vi "Pagina parametri.vi"() -> (6 "pagina out":i16)   [LabVIEW 2022 SP3]
uses:
  Labview/Globali.vi
panel:
  in  "230. 0":sgl min=0 format="%.2f"
  in  "226. 0":sgl min=0 format="%.2f"
  in  "Azzeramento \ntorsiometro (V)":sgl min=0 format="%.2f"
  in  "Carica da file":bool
  in  "Salva":bool
  in  "stop":bool
  out "Indicazioni":string
  out "Prodotto":string
  out "Testo allarmi":string caption="ALLARMI"
  out "Testo fase collaudo":string caption="FASE COLLAUDO"
  out "Testo segnalazioni":string caption="SEGNALAZIONI"
  out "Testo messaggi":string caption="MESSAGGI"
  out "Tipo pagina":string
  out "Picture":picture
  out "Versione SW":dbl=1.0 format="%.2f"
  out "Linea":string="CENTAURO"
  in  "8. 0":i16 min=0
  in  "12. 0":sgl min=0 format="%.2f"
  in  "16. 0":i16 min=0
  in  "22. 0":sgl min=0 format="%.2f"
  in  "26. 0":sgl min=0 format="%.2f"
  in  "32. 0":sgl min=0 format="%.2f"
  in  "36. 0":sgl min=0 format="%.2f"
  in  "44. 0":i16 min=0
  in  "50. 0":i16 min=0
  in  "56. 0":i16 min=0
  in  "62. 0":i16 min=0
  in  "68. 0":i16 min=0
  in  "72. 0":sgl min=0 format="%.2f"
  in  "76. 0":sgl min=0 format="%.2f"
  in  "80. 0":sgl min=0 format="%.2f"
  in  "84. 0":i16 min=0
  in  "88. 0":sgl min=0 format="%.2f"
  in  "92. 0":sgl min=0 format="%.2f"
  in  "96. 0":sgl min=0 format="%.2f"
  in  "100. 0":i16 min=0
  in  "104. 0":sgl min=0 format="%.2f"
  in  "108. 0":sgl min=0 format="%.2f"
  in  "112. 0":sgl min=0 format="%.2f"
  in  "116. 0":i16 min=0
  in  "120. 0":sgl min=0 format="%.2f"
  in  "124. 0":sgl min=0 format="%.2f"
  in  "128. 0":sgl min=0 format="%.2f"
  in  "134. 0":sgl min=0 format="%.2f"
  in  "138. 0":sgl min=0 format="%.2f"
  in  "144. 0":i16 min=0
  in  "148. 0":i16 min=0
  in  "154. 0":i16 min=0
  in  "160. 0":sgl min=0 format="%.2f"
  in  "164. 0":sgl min=0 format="%.2f"
  in  "168. 0":sgl min=0 format="%.2f"
  in  "172. 0":i16 min=0
  in  "176. 0":sgl min=0 format="%.2f"
  in  "180. 0":sgl min=0 format="%.2f"
  in  "184. 0":sgl min=0 format="%.2f"
  in  "190. 0":sgl min=0 format="%.2f"
  in  "194. 0":sgl min=0 format="%.2f"
  in  "200. 0":i16 min=0
  in  "206. 0":i16 min=0
  in  "212. 0":i16 min=0
  in  "20. 0":u16
  in  "30. 0":u16
  in  "40. 0":u16
  in  "42. 0":u16
  in  "48. 0":u16
  in  "54. 0":u16
  in  "60. 0":u16
  in  "66. 0":u16
  in  "132. 0":u16
  in  "142. 0":u16
  in  "152. 0":u16
  in  "158. 0":u16
  in  "188. 0":u16
  in  "198. 0":u16
  in  "204. 0":u16
  in  "210. 0":u16
  in  "216. 0":u16
  in  "218. 0":u16
  in  "NOME PRODOTTO":string
  out "error out":errorcluster
  in  "error in":errorcluster
  # "RISCALDAMENTO"
  # "FUNZIONAMENTO"
  # "Temperatura olio RP riscaldamento"
  # "Pressione ricircolo minima"
  # "Pressione gonfiaggio minima"
  # "Velocità motore riscaldamento"
  # "Pressione ricircolo massima"
  # "Pressione gonfiaggio massima"
  # "Tempo AAT riscaldamento"
  # "Velocità motore 1 funzionamento"
  # "Tempo stabilizzazione gonfiaggio"
  # "Pressione olio ricircolo minima"
  # "Temperatura olio 1 funzionamento"
  # "Vel. motore 4 funzionamento RP dx"
  # "K_VEL_MOT_MAN"
  # "Pressione olio ricircolo massima"
  # "Coppia 1 funzionamento minima"
  # "Velocità motore 4 funzionamento"
  # "Coppia 1 funzionamento massima"
  # "Tempo 4 funzionamento RP dx"
  # "Velocità motore 2 funzionamento"
  # "Vel. motore 4 funzionamento RP sx"
  # "INSERZIONE 1° ASSE"
  # "Temperatura olio 2 funzionamento"
  # "Tempo 4 funzionamento RP sx"
  # "Tempo pressurizzazione inserzione"
  # "Coppia 2 funzionamento minima"
  # "Temperatura olio 4 funzionamento"
  # "Pressurizzaz. inserz. asse minima"
  # "Coppia 2 funzionamento massima"
  # "Coppia 4 funzionamento minima"
  # "Pressurizzaz. inserz. asse massima"
  # "Velocità motore 3 funzionamento"
  # "Coppia 4 funzionamento massima"
  # "Tempo inserzione 1° asse"
  # "Temperatura olio 3 funzionamento"
  # "Velocità motore 5 funzionamento"
  # "Tempo disinserzione 1° asse"
  # "Coppia 3 funzionamento minima"
  # "Temperatura olio 5 funzionamento"
  # "Coppia 3 funzionamento massima"
  # "Coppia 5 funzionamento minima"
  # "Tempo gonfiaggio"
  # "Coppia 5 funzionamento massima"
  # "RODAGGIO"
  # "Perdita gonfiaggio"
  # "Velocità 1 motore rodaggio"
  # "PRESSURIZZAZIONE"
  # "PROT35"
  # "Tempo 1 rodaggio"
  # "Tempo pressurizzazione"
  # "Velocità motore PROT35"
  # "Velocità 2 motore rodaggio"
  # "Pressurizzazione minima"
  # "Tempo PROT35 sx"
  # "Tempo 2 rodaggio"
  # "Pressurizzazione massima"
  # "Tempo PROT35 dx"
  # "Velocità 3 motore rodaggio"
  # "Tempo stabilizzazione pressurizzaz."
  # "Tempo 3 rodaggio"
  # "Velocità pressurizzazione dx"
  # "Velocità 4 motore rodaggio"
  # "Tempo pressurizzazione dx"
  # "Tempo 4 rodaggio"
  # "Velocità pressurizzazione sx"
  # "Velocità 5 motore rodaggio"
  # "Tempo pressurizzazione sx"
  # "Temperatura olio rodaggio"
  # "Perdita pressurizzazione"
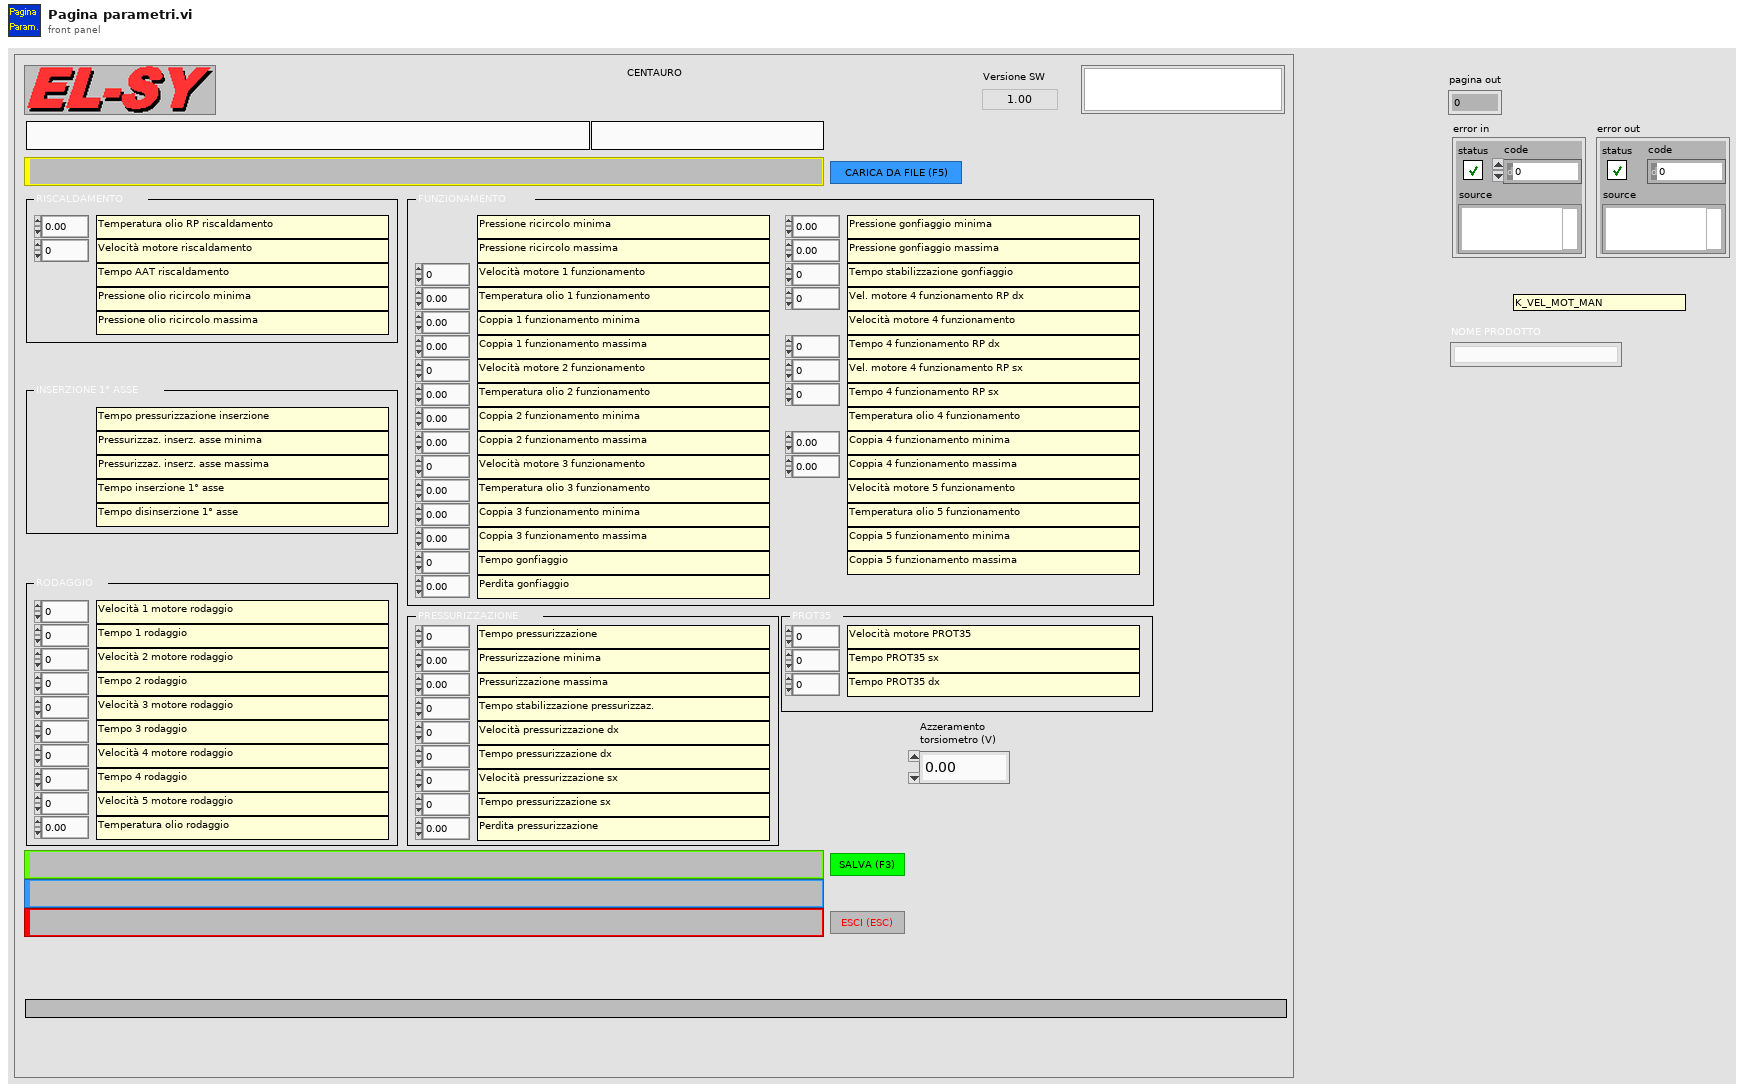
[diagram p1: front panel]
types:
  T1 = enum16{"open", "open or create", "create or replace", "create", "open (read only)"}
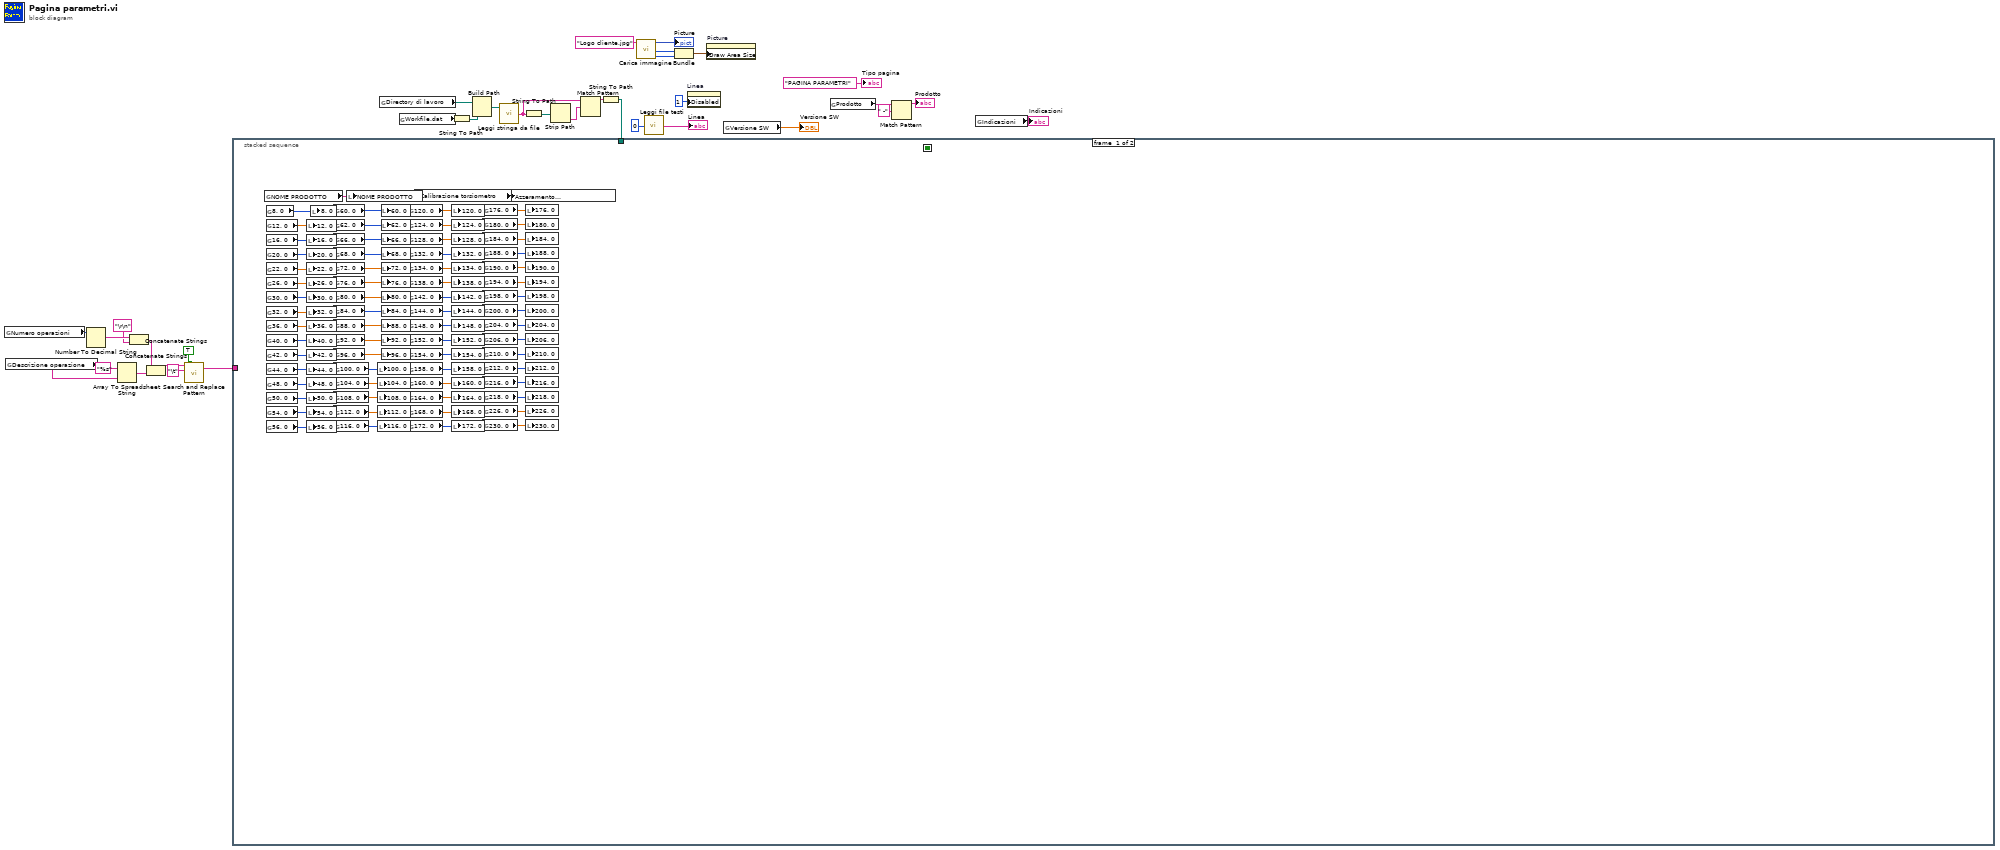
[diagram p0: block diagram]
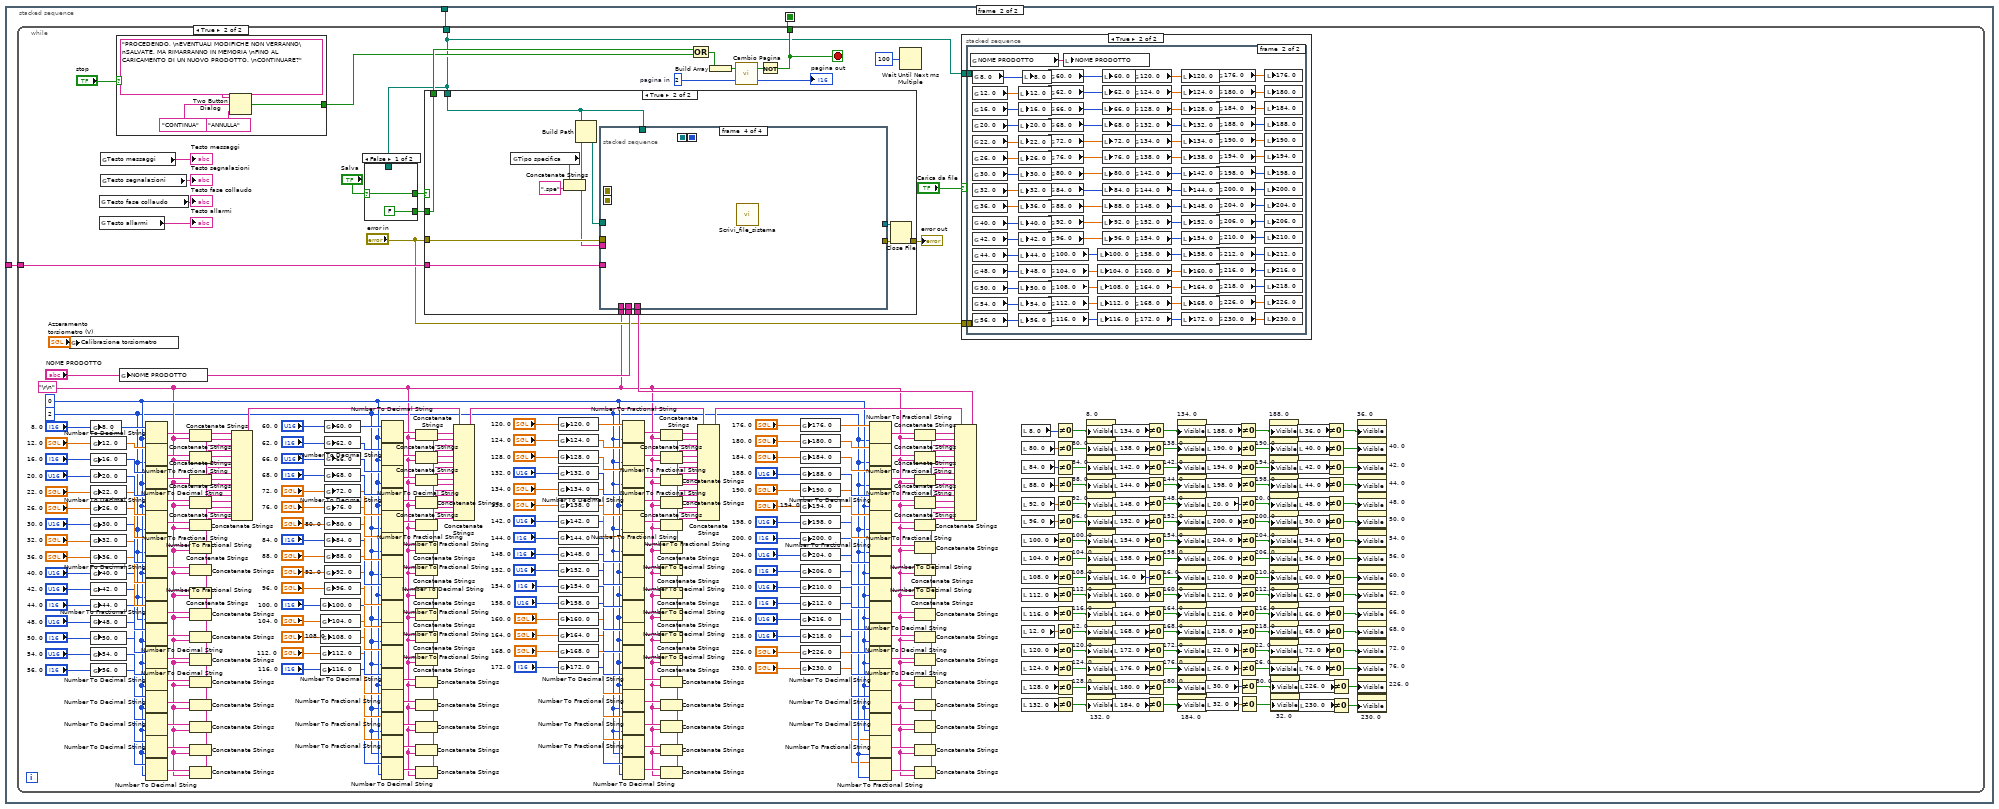
[diagram p2: hidden frame]
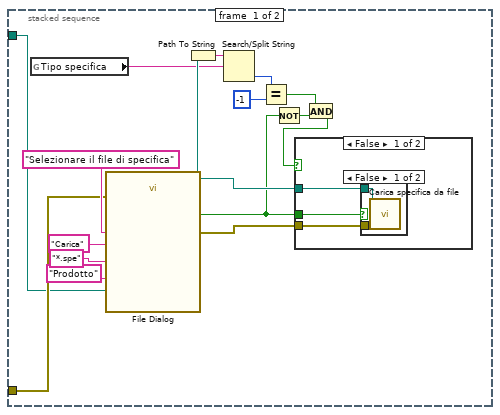
[diagram p4: hidden frame]
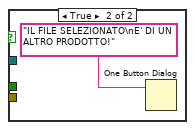
[diagram p6: hidden frame]
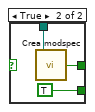
[diagram p8: hidden frame]
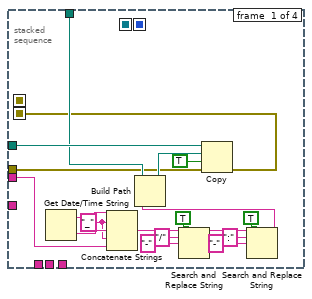
[diagram p10: hidden frame]
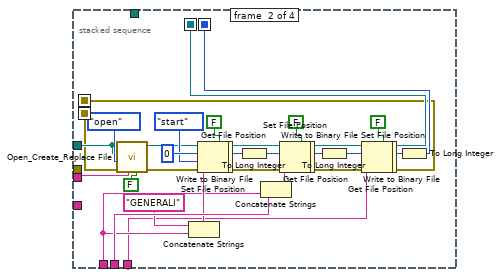
[diagram p11: hidden frame]
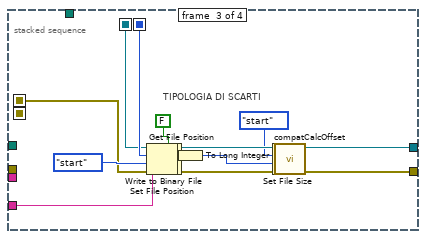
[diagram p12: hidden frame]
diagram:
  n1 = global read "Globali.vi" "Numero operazioni"() -> (w13:u16)
  n2 = global read "Globali.vi" "Descrizione operazione"() -> (w16:string[])
  n3 = Number To Decimal String(number=w13) -> (decimal integer string=w12:string)  [unwired: 1 in]
  n4 = Array To Spreadsheet String(array=w16, 3:"%s" ("format string")) -> (spreadsheet string=w15:string)  [unwired: 1 in]
  n5 = Concatenate Strings(w12, "\r\n" ("delimiter (Tab)")) -> (w11:string)
  n6 = Concatenate Strings(w11, w15) -> (w8:string)
  n7 = call <vilib>:"Search and Replace Pattern.vi"("string"=w8, "regular expression (\"\")"="\t" ("regular expression (\"\")"), "replace all? (F)"=TRUE) -> ("result string"=w9:string)  [unwired: 2 in, 1 out]
  n8 = global read "Globali.vi" "Directory di lavoro"() -> (w32:path)
  n9 = global read "Globali.vi" "Workfile.dat"() -> (w31:string)
  n10 = String To Path(string=w31) -> (path=w34:path)
  n11 = Build Path(base path=w32, name or relative path=w34) -> (appended path=w33:path)
  n12 = call "Leggi stringa da file.vi"("file path (dialog if empty)"=w33) -> ("character string"=w27:string)  [unwired: 5 in, 3 out]
  n13 = String To Path(string=w27) -> (path=w30:path)
  n14 = Strip Path(path=w30) -> (name=w29:string)  [unwired: 1 out]
  n15 = Match Pattern(string=w27, regular expression=w29) -> (before substring=w28:string)  [unwired: 1 in, 3 out]
  n16 = String To Path(string=w28) -> (path=w26:path)
  n17 = stacked-sequence {
    seq-local: [_ w102] -> [_ _]
    tunnel: w26 -> [_ w103]
    tunnel: w9 -> [_ w101]
    frame #0 {
      n18 = global read "Globali.vi" "NOME PRODOTTO"() -> (w100:string)
      n19 = global read "Globali.vi" "8. 0"() -> (w99:i16)
      n20 = global read "Globali.vi" "12. 0"() -> (w98:sgl)
      n21 = global read "Globali.vi" "16. 0"() -> (w97:i16)
      n22 = global read "Globali.vi" "20. 0"() -> (w96:u16)
      n23 = global read "Globali.vi" "22. 0"() -> (w95:sgl)
      n24 = global read "Globali.vi" "26. 0"() -> (w94:sgl)
      n25 = global read "Globali.vi" "30. 0"() -> (w93:u16)
      n26 = global read "Globali.vi" "32. 0"() -> (w92:sgl)
      n27 = global read "Globali.vi" "36. 0"() -> (w91:sgl)
      n28 = global read "Globali.vi" "40. 0"() -> (w90:u16)
      n29 = global read "Globali.vi" "42. 0"() -> (w89:u16)
      n30 = global read "Globali.vi" "44. 0"() -> (w88:i16)
      n31 = global read "Globali.vi" "48. 0"() -> (w87:u16)
      n32 = global read "Globali.vi" "50. 0"() -> (w86:i16)
      n33 = global read "Globali.vi" "54. 0"() -> (w85:u16)
      n34 = global read "Globali.vi" "56. 0"() -> (w84:i16)
      n35 = local write "12. 0"(w98) -> ()
      n36 = local write "16. 0"(w97) -> ()
      n37 = local write "20. 0"(w96) -> ()
      n38 = local write "22. 0"(w95) -> ()
      n39 = local write "26. 0"(w94) -> ()
      n40 = local write "30. 0"(w93) -> ()
      n41 = local write "32. 0"(w92) -> ()
      n42 = local write "36. 0"(w91) -> ()
      n43 = local write "40. 0"(w90) -> ()
      n44 = local write "42. 0"(w89) -> ()
      n45 = local write "44. 0"(w88) -> ()
      n46 = local write "48. 0"(w87) -> ()
      n47 = local write "50. 0"(w86) -> ()
      n48 = local write "54. 0"(w85) -> ()
      n49 = local write "56. 0"(w84) -> ()
      n50 = local write "8. 0"(w99) -> ()
      n51 = global read "Globali.vi" "60. 0"() -> (w83:u16)
      n52 = global read "Globali.vi" "62. 0"() -> (w82:i16)
      n53 = global read "Globali.vi" "66. 0"() -> (w81:u16)
      n54 = global read "Globali.vi" "68. 0"() -> (w80:i16)
      n55 = global read "Globali.vi" "72. 0"() -> (w79:sgl)
      n56 = global read "Globali.vi" "76. 0"() -> (w78:sgl)
      n57 = global read "Globali.vi" "80. 0"() -> (w77:sgl)
      n58 = global read "Globali.vi" "84. 0"() -> (w76:i16)
      n59 = global read "Globali.vi" "88. 0"() -> (w75:sgl)
      n60 = global read "Globali.vi" "92. 0"() -> (w74:sgl)
      n61 = global read "Globali.vi" "96. 0"() -> (w73:sgl)
      n62 = global read "Globali.vi" "100. 0"() -> (w72:i16)
      n63 = global read "Globali.vi" "104. 0"() -> (w71:sgl)
      n64 = global read "Globali.vi" "108. 0"() -> (w70:sgl)
      n65 = global read "Globali.vi" "112. 0"() -> (w69:sgl)
      n66 = global read "Globali.vi" "116. 0"() -> (w68:i16)
      n67 = local write "NOME PRODOTTO"(w100) -> ()
      n68 = local write "100. 0"(w72) -> ()
      n69 = local write "104. 0"(w71) -> ()
      n70 = local write "108. 0"(w70) -> ()
      n71 = local write "112. 0"(w69) -> ()
      n72 = local write "116. 0"(w68) -> ()
      n73 = local write "60. 0"(w83) -> ()
      n74 = local write "62. 0"(w82) -> ()
      n75 = local write "66. 0"(w81) -> ()
      n76 = local write "68. 0"(w80) -> ()
      n77 = local write "72. 0"(w79) -> ()
      n78 = local write "76. 0"(w78) -> ()
      n79 = local write "80. 0"(w77) -> ()
      n80 = local write "84. 0"(w76) -> ()
      n81 = local write "88. 0"(w75) -> ()
      n82 = local write "92. 0"(w74) -> ()
      n83 = local write "96. 0"(w73) -> ()
      n84 = global read "Globali.vi" "120. 0"() -> (w67:sgl)
      n85 = global read "Globali.vi" "124. 0"() -> (w66:sgl)
      n86 = global read "Globali.vi" "128. 0"() -> (w65:sgl)
      n87 = global read "Globali.vi" "132. 0"() -> (w64:u16)
      n88 = global read "Globali.vi" "134. 0"() -> (w63:sgl)
      n89 = global read "Globali.vi" "138. 0"() -> (w62:sgl)
      n90 = global read "Globali.vi" "142. 0"() -> (w61:u16)
      n91 = global read "Globali.vi" "144. 0"() -> (w60:i16)
      n92 = global read "Globali.vi" "148. 0"() -> (w59:i16)
      n93 = global read "Globali.vi" "152. 0"() -> (w58:u16)
      n94 = global read "Globali.vi" "154. 0"() -> (w57:i16)
      n95 = global read "Globali.vi" "158. 0"() -> (w56:u16)
      n96 = global read "Globali.vi" "160. 0"() -> (w55:sgl)
      n97 = global read "Globali.vi" "164. 0"() -> (w54:sgl)
      n98 = global read "Globali.vi" "168. 0"() -> (w53:sgl)
      n99 = global read "Globali.vi" "172. 0"() -> (w52:i16)
      n100 = global read "Globali.vi" "Calibrazione torsiometro"() -> (w37:sgl)
      n101 = local write "120. 0"(w67) -> ()
      n102 = local write "124. 0"(w66) -> ()
      n103 = local write "128. 0"(w65) -> ()
      n104 = local write "132. 0"(w64) -> ()
      n105 = local write "134. 0"(w63) -> ()
      n106 = local write "138. 0"(w62) -> ()
      n107 = local write "142. 0"(w61) -> ()
      n108 = local write "144. 0"(w60) -> ()
      n109 = local write "148. 0"(w59) -> ()
      n110 = local write "152. 0"(w58) -> ()
      n111 = local write "154. 0"(w57) -> ()
      n112 = local write "158. 0"(w56) -> ()
      n113 = local write "160. 0"(w55) -> ()
      n114 = local write "164. 0"(w54) -> ()
      n115 = local write "168. 0"(w53) -> ()
      n116 = local write "172. 0"(w52) -> ()
      n117 = global read "Globali.vi" "176. 0"() -> (w51:sgl)
      n118 = global read "Globali.vi" "180. 0"() -> (w50:sgl)
      n119 = global read "Globali.vi" "184. 0"() -> (w49:sgl)
      n120 = global read "Globali.vi" "188. 0"() -> (w48:u16)
      n121 = global read "Globali.vi" "190. 0"() -> (w47:sgl)
      n122 = global read "Globali.vi" "194. 0"() -> (w46:sgl)
      n123 = global read "Globali.vi" "198. 0"() -> (w45:u16)
      n124 = global read "Globali.vi" "200. 0"() -> (w44:i16)
      n125 = global read "Globali.vi" "204. 0"() -> (w43:u16)
      n126 = global read "Globali.vi" "206. 0"() -> (w42:i16)
      n127 = global read "Globali.vi" "210. 0"() -> (w41:u16)
      n128 = global read "Globali.vi" "212. 0"() -> (w40:i16)
      n129 = global read "Globali.vi" "216. 0"() -> (w39:u16)
      n130 = global read "Globali.vi" "218. 0"() -> (w38:u16)
      n131 = global read "Globali.vi" "226. 0"() -> (w35:sgl)
      n132 = global read "Globali.vi" "230. 0"() -> (w36:sgl)
      n133 = local write "Azzeramento \ntorsiometro (V)"(w37) -> ()
      n134 = local write "176. 0"(w51) -> ()
      n135 = local write "180. 0"(w50) -> ()
      n136 = local write "184. 0"(w49) -> ()
      n137 = local write "188. 0"(w48) -> ()
      n138 = local write "190. 0"(w47) -> ()
      n139 = local write "194. 0"(w46) -> ()
      n140 = local write "198. 0"(w45) -> ()
      n141 = local write "200. 0"(w44) -> ()
      n142 = local write "204. 0"(w43) -> ()
      n143 = local write "206. 0"(w42) -> ()
      n144 = local write "210. 0"(w41) -> ()
      n145 = local write "212. 0"(w40) -> ()
      n146 = local write "216. 0"(w39) -> ()
      n147 = local write "218. 0"(w38) -> ()
      n148 = local write "226. 0"(w35) -> ()
      n149 = local write "230. 0"(w36) -> ()
    }
    frame #1 {
      n150 = while {
        tunnel: w103 -> [w241]
        tunnel: [w254] -> w102
        tunnel: w101 -> [w446]
        stop <- w254 stop-if-true
        w110 = i16 2 ("width (-)")
        w255 = i16 0 ("width (-)")
        w113 = "\r\n"
        w453 = u8 2  # pagina in
        n151 = global write "Globali.vi" "Calibrazione torsiometro"("Azzeramento \ntorsiometro (V)") -> ()
        n152 = global write "Globali.vi" "8. 0"("8. 0") -> ()
        n153 = global write "Globali.vi" "12. 0"("12. 0") -> ()
        n154 = global write "Globali.vi" "16. 0"("16. 0") -> ()
        n155 = global write "Globali.vi" "20. 0"("20. 0") -> ()
        n156 = global write "Globali.vi" "22. 0"("22. 0") -> ()
        n157 = global write "Globali.vi" "26. 0"("26. 0") -> ()
        n158 = global write "Globali.vi" "30. 0"("30. 0") -> ()
        n159 = global write "Globali.vi" "32. 0"("32. 0") -> ()
        n160 = global write "Globali.vi" "36. 0"("36. 0") -> ()
        n161 = global write "Globali.vi" "40. 0"("40. 0") -> ()
        n162 = global write "Globali.vi" "42. 0"("42. 0") -> ()
        n163 = global write "Globali.vi" "44. 0"("44. 0") -> ()
        n164 = global write "Globali.vi" "48. 0"("48. 0") -> ()
        n165 = global write "Globali.vi" "50. 0"("50. 0") -> ()
        n166 = global write "Globali.vi" "54. 0"("54. 0") -> ()
        n167 = global write "Globali.vi" "56. 0"("56. 0") -> ()
        n168 = global read "Globali.vi" "Testo fase collaudo"() -> (→"Testo fase collaudo":string)
        n169 = global read "Globali.vi" "Testo allarmi"() -> (→"Testo allarmi":string)
        n170 = global read "Globali.vi" "Testo messaggi"() -> (→"Testo messaggi":string)
        n171 = global read "Globali.vi" "Testo segnalazioni"() -> (→"Testo segnalazioni":string)
        n172 = case shown="True" "stop" {
          selector: "stop" -> [w544 _]
          tunnel: [w544 w548] -> w245
          frame False {
          }
          frame True {
            n173 = Two Button Dialog(message="PROCEDENDO, \nEVENTUALI MODIFICHE NON VERRANNO\nSALVATE, MA RIMARRANNO IN MEMORIA \nFINO AL CARICAMENTO DI UN NUOVO PRODOTTO. \nCONTINUARE?", 1:"ANNULLA" ("F button name (\"Cancel\")"), 2:"CONTINUA" ("T button name (\"OK\")")) -> (T button?=w548:bool)
          }
        }
        n174 = global write "Globali.vi" "NOME PRODOTTO"("NOME PRODOTTO") -> ()
        n175 = Number To Decimal String(number="8. 0", width (-)=w255) -> (decimal integer string=w383:string)
        n176 = Number To Fractional String(number="12. 0", precision (6)=w110) -> (F-format string=w381:string)  [unwired: 2 in]
        n177 = Number To Decimal String(number="16. 0", width (-)=w255) -> (decimal integer string=w323:string)
        n178 = Number To Decimal String(number="20. 0", width (-)=w255) -> (decimal integer string=w380:string)
        n179 = Number To Fractional String(number="22. 0", precision (6)=w110) -> (F-format string=w379:string)  [unwired: 2 in]
        n180 = Number To Fractional String(number="26. 0", precision (6)=w110) -> (F-format string=w378:string)  [unwired: 2 in]
        n181 = Number To Decimal String(number="30. 0", width (-)=w255) -> (decimal integer string=w377:string)
        n182 = Number To Fractional String(number="32. 0", precision (6)=w110) -> (F-format string=w376:string)  [unwired: 2 in]
        n183 = Number To Fractional String(number="36. 0", precision (6)=w110) -> (F-format string=w375:string)  [unwired: 2 in]
        n184 = Number To Decimal String(number="40. 0", width (-)=w255) -> (decimal integer string=w374:string)
        n185 = Number To Decimal String(number="42. 0", width (-)=w255) -> (decimal integer string=w373:string)
        n186 = Number To Decimal String(number="44. 0", width (-)=w255) -> (decimal integer string=w372:string)
        n187 = Number To Decimal String(number="48. 0", width (-)=w255) -> (decimal integer string=w371:string)
        n188 = Number To Decimal String(number="50. 0", width (-)=w255) -> (decimal integer string=w370:string)
        n189 = Number To Decimal String(number="54. 0", width (-)=w255) -> (decimal integer string=w369:string)
        n190 = Number To Decimal String(number="56. 0", width (-)=w255) -> (decimal integer string=w382:string)
        n191 = Concatenate Strings(w383, w113) -> (w321:string)
        n192 = Concatenate Strings(w381, w113) -> (w320:string)
        n193 = Concatenate Strings(w323, w113) -> (w319:string)
        n194 = Concatenate Strings(w380, w113) -> (w318:string)
        n195 = Concatenate Strings(w379, w113) -> (w317:string)
        n196 = Concatenate Strings(w378, w113) -> (w316:string)
        n197 = Concatenate Strings(w377, w113) -> (w315:string)
        n198 = Concatenate Strings(w376, w113) -> (w314:string)
        n199 = Concatenate Strings(w375, w113) -> (w313:string)
        n200 = Concatenate Strings(w374, w113) -> (w312:string)
        n201 = Concatenate Strings(w373, w113) -> (w311:string)
        n202 = Concatenate Strings(w372, w113) -> (w310:string)
        n203 = Concatenate Strings(w371, w113) -> (w309:string)
        n204 = Concatenate Strings(w370, w113) -> (w308:string)
        n205 = Concatenate Strings(w369, w113) -> (w307:string)
        n206 = Concatenate Strings(w382, w113) -> (w306:string)
        n207 = Concatenate Strings(w321, w320, w319, w318, w317, w316, w315, w314, w313, w312, w311, w310, w309, w308, w307, w306) -> (w305:string)
        n208 = global write "Globali.vi" "100. 0"("100. 0") -> ()
        n209 = global write "Globali.vi" "104. 0"("104. 0") -> ()
        n210 = global write "Globali.vi" "108. 0"("108. 0") -> ()
        n211 = global write "Globali.vi" "112. 0"("112. 0") -> ()
        n212 = global write "Globali.vi" "116. 0"("116. 0") -> ()
        n213 = global write "Globali.vi" "60. 0"("60. 0") -> ()
        n214 = global write "Globali.vi" "62. 0"("62. 0") -> ()
        n215 = global write "Globali.vi" "66. 0"("66. 0") -> ()
        n216 = global write "Globali.vi" "68. 0"("68. 0") -> ()
        n217 = global write "Globali.vi" "72. 0"("72. 0") -> ()
        n218 = global write "Globali.vi" "76. 0"("76. 0") -> ()
        n219 = global write "Globali.vi" "80. 0"("80. 0") -> ()
        n220 = global write "Globali.vi" "84. 0"("84. 0") -> ()
        n221 = global write "Globali.vi" "88. 0"("88. 0") -> ()
        n222 = global write "Globali.vi" "92. 0"("92. 0") -> ()
        n223 = global write "Globali.vi" "96. 0"("96. 0") -> ()
        n224 = case shown="False" "Salva" {
          selector: "Salva" -> [w550 _]
          tunnel: [w550 w553] -> w448
          tunnel: w241 -> [_ w552]
          tunnel: [FALSE TRUE] -> w247
          frame False {
          }
          frame True {
            n225 = call "Crea modspec.vi"("base path"=w552) -> ("Salva s/n"=w553:bool)  [unwired: 4 in]
          }
        }
        n226 = Number To Decimal String(number="60. 0", width (-)=w255) -> (decimal integer string=w368:string)
        n227 = Number To Decimal String(number="62. 0", width (-)=w255) -> (decimal integer string=w367:string)
        n228 = Number To Decimal String(number="66. 0", width (-)=w255) -> (decimal integer string=w366:string)
        n229 = Number To Decimal String(number="68. 0", width (-)=w255) -> (decimal integer string=w365:string)
        n230 = Number To Fractional String(number="72. 0", precision (6)=w110) -> (F-format string=w364:string)  [unwired: 2 in]
        n231 = Number To Fractional String(number="76. 0", precision (6)=w110) -> (F-format string=w363:string)  [unwired: 2 in]
        n232 = Number To Fractional String(number="80. 0", precision (6)=w110) -> (F-format string=w362:string)  [unwired: 2 in]
        n233 = Number To Decimal String(number="84. 0", width (-)=w255) -> (decimal integer string=w361:string)
        n234 = Number To Fractional String(number="88. 0", precision (6)=w110) -> (F-format string=w360:string)  [unwired: 2 in]
        n235 = Number To Fractional String(number="92. 0", precision (6)=w110) -> (F-format string=w359:string)  [unwired: 2 in]
        n236 = Number To Fractional String(number="96. 0", precision (6)=w110) -> (F-format string=w358:string)  [unwired: 2 in]
        n237 = Number To Decimal String(number="100. 0", width (-)=w255) -> (decimal integer string=w357:string)
        n238 = Number To Fractional String(number="104. 0", precision (6)=w110) -> (F-format string=w356:string)  [unwired: 2 in]
        n239 = Number To Fractional String(number="108. 0", precision (6)=w110) -> (F-format string=w322:string)  [unwired: 2 in]
        n240 = Number To Fractional String(number="112. 0", precision (6)=w110) -> (F-format string=w355:string)  [unwired: 2 in]
        n241 = Number To Decimal String(number="116. 0", width (-)=w255) -> (decimal integer string=w354:string)
        n242 = Concatenate Strings(w368, w113) -> (w304:string)
        n243 = Concatenate Strings(w367, w113) -> (w303:string)
        n244 = Concatenate Strings(w366, w113) -> (w302:string)
        n245 = Concatenate Strings(w365, w113) -> (w301:string)
        n246 = Concatenate Strings(w364, w113) -> (w300:string)
        n247 = Concatenate Strings(w363, w113) -> (w299:string)
        n248 = Concatenate Strings(w362, w113) -> (w298:string)
        n249 = Concatenate Strings(w361, w113) -> (w297:string)
        n250 = Concatenate Strings(w360, w113) -> (w296:string)
        n251 = Concatenate Strings(w359, w113) -> (w295:string)
        n252 = Concatenate Strings(w358, w113) -> (w294:string)
        n253 = Concatenate Strings(w357, w113) -> (w293:string)
        n254 = Concatenate Strings(w356, w113) -> (w292:string)
        n255 = Concatenate Strings(w322, w113) -> (w291:string)
        n256 = Concatenate Strings(w355, w113) -> (w290:string)
        n257 = Concatenate Strings(w354, w113) -> (w289:string)
        n258 = Concatenate Strings(w305, w304, w303, w302, w301, w300, w299, w298, w297, w296, w295, w294, w293, w292, w291, w290, w289) -> (w288:string)
        n259 = global write "Globali.vi" "120. 0"("120. 0") -> ()
        n260 = global write "Globali.vi" "124. 0"("124. 0") -> ()
        n261 = global write "Globali.vi" "128. 0"("128. 0") -> ()
        n262 = global write "Globali.vi" "132. 0"("132. 0") -> ()
        n263 = global write "Globali.vi" "134. 0"("134. 0") -> ()
        n264 = global write "Globali.vi" "138. 0"("138. 0") -> ()
        n265 = global write "Globali.vi" "142. 0"("142. 0") -> ()
        n266 = global write "Globali.vi" "144. 0"("144. 0") -> ()
        n267 = global write "Globali.vi" "148. 0"("148. 0") -> ()
        n268 = global write "Globali.vi" "152. 0"("152. 0") -> ()
        n269 = global write "Globali.vi" "154. 0"("154. 0") -> ()
        n270 = global write "Globali.vi" "158. 0"("158. 0") -> ()
        n271 = global write "Globali.vi" "160. 0"("160. 0") -> ()
        n272 = global write "Globali.vi" "164. 0"("164. 0") -> ()
        n273 = global write "Globali.vi" "168. 0"("168. 0") -> ()
        n274 = global write "Globali.vi" "172. 0"("172. 0") -> ()
        n275 = Number To Fractional String(number="120. 0", precision (6)=w110) -> (F-format string=w353:string)  [unwired: 2 in]
        n276 = Number To Fractional String(number="124. 0", precision (6)=w110) -> (F-format string=w352:string)  [unwired: 2 in]
        n277 = Number To Fractional String(number="128. 0", precision (6)=w110) -> (F-format string=w351:string)  [unwired: 2 in]
        n278 = Number To Decimal String(number="132. 0", width (-)=w255) -> (decimal integer string=w350:string)
        n279 = Number To Fractional String(number="134. 0", precision (6)=w110) -> (F-format string=w349:string)  [unwired: 2 in]
        n280 = Number To Fractional String(number="138. 0", precision (6)=w110) -> (F-format string=w348:string)  [unwired: 2 in]
        n281 = Number To Decimal String(number="142. 0", width (-)=w255) -> (decimal integer string=w347:string)
        n282 = Number To Decimal String(number="144. 0", width (-)=w255) -> (decimal integer string=w346:string)
        n283 = Number To Decimal String(number="148. 0", width (-)=w255) -> (decimal integer string=w345:string)
        n284 = Number To Decimal String(number="152. 0", width (-)=w255) -> (decimal integer string=w344:string)
        n285 = Number To Decimal String(number="154. 0", width (-)=w255) -> (decimal integer string=w343:string)
        n286 = Number To Decimal String(number="158. 0", width (-)=w255) -> (decimal integer string=w342:string)
        n287 = Number To Fractional String(number="160. 0", precision (6)=w110) -> (F-format string=w341:string)  [unwired: 2 in]
        n288 = Number To Fractional String(number="164. 0", precision (6)=w110) -> (F-format string=w340:string)  [unwired: 2 in]
        n289 = Number To Fractional String(number="168. 0", precision (6)=w110) -> (F-format string=w339:string)  [unwired: 2 in]
        n290 = Number To Decimal String(number="172. 0", width (-)=w255) -> (decimal integer string=w338:string)
        n291 = Concatenate Strings(w353, w113) -> (w287:string)
        n292 = Concatenate Strings(w352, w113) -> (w286:string)
        n293 = Concatenate Strings(w351, w113) -> (w285:string)
        n294 = Concatenate Strings(w350, w113) -> (w284:string)
        n295 = Concatenate Strings(w349, w113) -> (w283:string)
        n296 = Concatenate Strings(w348, w113) -> (w282:string)
        n297 = Concatenate Strings(w347, w113) -> (w281:string)
        n298 = Concatenate Strings(w346, w113) -> (w280:string)
        n299 = Concatenate Strings(w345, w113) -> (w279:string)
        n300 = Concatenate Strings(w344, w113) -> (w278:string)
        n301 = Concatenate Strings(w343, w113) -> (w277:string)
        n302 = Concatenate Strings(w342, w113) -> (w276:string)
        n303 = Concatenate Strings(w341, w113) -> (w275:string)
        n304 = Concatenate Strings(w340, w113) -> (w274:string)
        n305 = Concatenate Strings(w339, w113) -> (w273:string)
        n306 = Concatenate Strings(w338, w113) -> (w272:string)
        n307 = Concatenate Strings(w288, w287, w286, w285, w284, w283, w282, w281, w280, w279, w278, w277, w276, w275, w274, w273, w272) -> (w271:string)
        n308 = global write "Globali.vi" "176. 0"("176. 0") -> ()
        n309 = global write "Globali.vi" "180. 0"("180. 0") -> ()
        n310 = global write "Globali.vi" "184. 0"("184. 0") -> ()
        n311 = global write "Globali.vi" "188. 0"("188. 0") -> ()
        n312 = global write "Globali.vi" "190. 0"("190. 0") -> ()
        n313 = global write "Globali.vi" "194. 0"("194. 0") -> ()
        n314 = global write "Globali.vi" "198. 0"("198. 0") -> ()
        n315 = global write "Globali.vi" "200. 0"("200. 0") -> ()
        n316 = global write "Globali.vi" "204. 0"("204. 0") -> ()
        n317 = global write "Globali.vi" "206. 0"("206. 0") -> ()
        n318 = global write "Globali.vi" "210. 0"("210. 0") -> ()
        n319 = global write "Globali.vi" "212. 0"("212. 0") -> ()
        n320 = global write "Globali.vi" "216. 0"("216. 0") -> ()
        n321 = global write "Globali.vi" "218. 0"("218. 0") -> ()
        n322 = global write "Globali.vi" "226. 0"("226. 0") -> ()
        n323 = global write "Globali.vi" "230. 0"("230. 0") -> ()
        n324 = Number To Fractional String(number="176. 0", precision (6)=w110) -> (F-format string=w337:string)  [unwired: 2 in]
        n325 = Number To Fractional String(number="180. 0", precision (6)=w110) -> (F-format string=w336:string)  [unwired: 2 in]
        n326 = Number To Fractional String(number="184. 0", precision (6)=w110) -> (F-format string=w335:string)  [unwired: 2 in]
        n327 = Number To Decimal String(number="188. 0", width (-)=w255) -> (decimal integer string=w334:string)
        n328 = Number To Fractional String(number="190. 0", precision (6)=w110) -> (F-format string=w333:string)  [unwired: 2 in]
        n329 = Number To Fractional String(number="194. 0", precision (6)=w110) -> (F-format string=w332:string)  [unwired: 2 in]
        n330 = Number To Decimal String(number="198. 0", width (-)=w255) -> (decimal integer string=w331:string)
        n331 = Number To Decimal String(number="200. 0", width (-)=w255) -> (decimal integer string=w330:string)
        n332 = Number To Decimal String(number="204. 0", width (-)=w255) -> (decimal integer string=w329:string)
        n333 = Number To Decimal String(number="206. 0", width (-)=w255) -> (decimal integer string=w328:string)
        n334 = Number To Decimal String(number="210. 0", width (-)=w255) -> (decimal integer string=w327:string)
        n335 = Number To Decimal String(number="212. 0", width (-)=w255) -> (decimal integer string=w326:string)
        n336 = Number To Decimal String(number="216. 0", width (-)=w255) -> (decimal integer string=w325:string)
        n337 = Number To Decimal String(number="218. 0", width (-)=w255) -> (decimal integer string=w324:string)
        n338 = Number To Fractional String(number="226. 0", precision (6)=w110) -> (F-format string=w114:string)  [unwired: 2 in]
        n339 = Number To Fractional String(number="230. 0", precision (6)=w110) -> (F-format string=w115:string)  [unwired: 2 in]
        n340 = Wait Until Next ms Multiple(millisecond multiple=u32 100) -> ()  [unwired: 1 out]
        n341 = Concatenate Strings(w337, w113) -> (w270:string)
        n342 = Concatenate Strings(w336, w113) -> (w269:string)
        n343 = Concatenate Strings(w335, w113) -> (w268:string)
        n344 = Concatenate Strings(w334, w113) -> (w267:string)
        n345 = Concatenate Strings(w333, w113) -> (w266:string)
        n346 = Concatenate Strings(w332, w113) -> (w265:string)
        n347 = Concatenate Strings(w331, w113) -> (w264:string)
        n348 = Concatenate Strings(w330, w113) -> (w263:string)
        n349 = Concatenate Strings(w329, w113) -> (w262:string)
        n350 = Concatenate Strings(w328, w113) -> (w261:string)
        n351 = Concatenate Strings(w327, w113) -> (w260:string)
        n352 = Concatenate Strings(w326, w113) -> (w259:string)
        n353 = Concatenate Strings(w325, w113) -> (w258:string)
        n354 = Concatenate Strings(w324, w113) -> (w257:string)
        n355 = Concatenate Strings(w114, w113) -> (w112:string)
        n356 = Concatenate Strings(w115, w113) -> (w111:string)
        n357 = Concatenate Strings(w271, w270, w269, w268, w267, w266, w265, w264, w263, w262, w261, w260, w259, w258, w257, w112, w111) -> (w256:string)
        n358 = case shown="True" w448 {
          tunnel: "error in" -> [w555 w558]
          tunnel: [w555 w569] -> w450
          tunnel: "NOME PRODOTTO" -> [_ w568]
          tunnel: w256 -> [_ w567]
          tunnel: w241 -> [_ w556]
          tunnel: w446 -> [_ w562]
          tunnel: w113 -> [_ w561]
          tunnel: [w554 w560] -> w248
          tunnel: w247 -> [w554 w560]
          frame False {
          }
          frame True {
            n359 = global read "Globali.vi" "Tipo specifica"() -> (w566:string)
            n360 = Concatenate Strings(w566, ".spe" ("string")) -> (w557:string)
            n361 = Build Path(base path=w556, name or relative path=w557) -> (appended path=w559:path)
            n362 = stacked-sequence {
              seq-local: [_ w598 _ _] -> [_ _ w641 _]
              seq-local: [_ w600 _ _] -> [_ _ w640 _]
              seq-local: [_ w599 _ _] -> [_ _ w630 _]
              seq-local: [w579 _ _ _] -> [_ w589 _ _]
              tunnel: [_ _ w645 _] -> w564
              tunnel: [_ _ w644 _] -> w563
              tunnel: w568 -> [_ w621 _ _]
              tunnel: w567 -> [_ w596 _ _]
              tunnel: w561 -> [_ w597 _ _]
              tunnel: w562 -> [_ _ w648 _]
              tunnel: w559 -> [w588 w591 _ _]
              tunnel: w558 -> [w580 _ _ _]
              tunnel: w557 -> [w584 w590 _ _]
              tunnel: w556 -> [w581 _ _ _]
              frame #0 {
                w585 = "_" ("string")
                n363 = Get Date/Time String() -> (date string=w587:string, time string=w586:string)  [unwired: 3 in]
                n364 = Concatenate Strings(w587, w585, w586, w585, w584) -> (w578:string)
                n365 = Search and Replace String(replace all?=TRUE ("replace all? (F)"), input string=w578, search string="/", replace string="-" ("replace string (\"\")")) -> (result string=w571:string)  [unwired: 4 in, 3 out]
                n366 = Search and Replace String(replace all?=TRUE ("replace all? (F)"), input string=w571, search string=":", replace string="-" ("replace string (\"\")")) -> (result string=w570:string)  [unwired: 4 in, 3 out]
                n367 = Build Path(base path=w581, name or relative path=w570) -> (appended path=w583:path)
                n368 = Copy(8:w580, 9:TRUE ("overwrite (F)"), 10:w583, 11:w588) -> (0:w579:errorcluster)  [unwired: 1 in, 2 out]
              }
              frame #1 {
                n369 = call <vilib>:"Open_Create_Replace File.vi"("advisory dialog? (display:T)"=FALSE, "default name"=w590, "error in (no error)"=w589, "function (open:0)"=T1."open", "start path  (Not A Path)"=w591, "file path"=w591) -> ("error out"=w593:errorcluster, "refnum"=w592:refnum<file>)  [unwired: 2 in, 2 out]
                n370 = Concatenate Strings("GENERALI" ("string"), w597) -> (w618:string)
                n371 = Set File Position(offset (in bytes) (0)=0 ("pos offset (0)"), refnum=w592, from (0:start)=enum16{"start", "end", "current"}."start" ("pos mode (0:2)"), error in=w593) -> (refnum out=w617:refnum<file>, error out=w616:errorcluster)
                n372 = Write to Binary File(file (use dialog)=w617, data=w618, error in=w616, 5:FALSE ("prepend array or string size? (T)")) -> (refnum out=w615:refnum<file>, error out=w614:errorcluster)  [unwired: 2 in, 1 out]
                n373 = Get File Position(4:w614, 7:w615) -> (0:w627:errorcluster, 2:w613:i64, 3:w623:refnum<file>)
                n374 = To Long Integer(number=w613) -> (32bit integer=w625:i32)
                n375 = Concatenate Strings(w621, w597) -> (w620:string)
                n376 = Set File Position(offset (in bytes) (0)=w625, refnum=w623, error in=w627) -> (refnum out=w607:refnum<file>, error out=w606:errorcluster)  [unwired: 1 in]
                n377 = Write to Binary File(file (use dialog)=w607, data=w620, error in=w606, 5:FALSE ("prepend array or string size? (T)")) -> (refnum out=w605:refnum<file>, error out=w604:errorcluster)  [unwired: 2 in, 1 out]
                n378 = Get File Position(4:w604, 7:w605) -> (0:w626:errorcluster, 2:w603:i64, 3:w622:refnum<file>)
                n379 = To Long Integer(number=w603) -> (32bit integer=w624:i32)
                n380 = Set File Position(offset (in bytes) (0)=w624, refnum=w622, error in=w626) -> (refnum out=w611:refnum<file>, error out=w610:errorcluster)  [unwired: 1 in]
                n381 = Write to Binary File(file (use dialog)=w611, data=w596, error in=w610, 5:FALSE ("prepend array or string size? (T)")) -> (refnum out=w601:refnum<file>, error out=w598:errorcluster)  [unwired: 2 in, 1 out]
                n382 = Get File Position(4:w598, 7:w601) -> (2:w609:i64, 3:w599:refnum<file>)  [unwired: 1 out]
                n383 = To Long Integer(number=w609) -> (32bit integer=w600:i32)
              }
              frame #2 {
                # "TIPOLOGIA DI SCARTI"
                n384 = Set File Position(offset (in bytes) (0)=w640, refnum=w630, from (0:start)=enum16{"start", "end", "current"}."start" ("pos mode (0:2)"), error in=w641) -> (refnum out=w636:refnum<file>, error out=w635:errorcluster)
                n385 = Write to Binary File(file (use dialog)=w636, data=w648, error in=w635, 5:FALSE ("prepend array or string size? (T)")) -> (refnum out=w634:refnum<file>, error out=w633:errorcluster)  [unwired: 2 in, 1 out]
                n386 = Get File Position(4:w633, 7:w634) -> (0:w646:errorcluster, 2:w632:i64, 3:w647:refnum<file>)
                n387 = To Long Integer(number=w632) -> (32bit integer=w643:i32)
                n388 = call <vilib>:"compatCalcOffset.vi"("error in"=w646, "pos offset (0)"=w643, "pos mode (0:1)"=enum16{"start", "end", "current"}."start", "refnum"=w647) -> ("error out"=w639:errorcluster, "offset"=w638:i32, "dup refnum"=w637:refnum<file>)  [unwired: 5 in]
                n389 = Set File Size(4:w639, 6:w638, 7:w637) -> (0:w645:errorcluster, 3:w644:refnum<file>)
              }
              frame #3 {
                n390 = call "Scrivi_file_sistema.vi"() -> ()  [unwired: 8 in]
              }
            }
            n391 = Close File(refnum=w563, error in=w564) -> (error out=w569:errorcluster)  [unwired: 1 out]
          }
        }
        "error out" <- w450
        n392 = Or(x=w248, y=w245) -> (x .or. y?=w249:bool)
        n393 = Build Array(w249) -> (w454:bool[])
        n394 = call "Cambio Pagina.vi"("pagina in"=w453, "pulsanti"=w454) -> ("pagina out"=→"pagina out":u8, "premuto"=w447:bool)
        n395 = Not(x=w447) -> (.not. x?=w254:bool)
        n396 = case shown="True" "Carica da file" {
          tunnel: "error in" -> [_ w456]
          tunnel: w241 -> [_ w455]
          frame False {
          }
          frame True {
            n397 = stacked-sequence {
              tunnel: w456 -> [w467 _]
              tunnel: w455 -> [w466 _]
              frame #0 {
                n398 = global read "Globali.vi" "Tipo specifica"() -> (w463:string)
                n399 = call "File Dialog"("start path"=w466, "prompt"="Selezionare il file di specifica", "button label"="Carica", "error in"=w467, "pattern (all files)"="*.spe", "pattern label"="Prodotto") -> ("selected path"=w465:path, "cancelled"=w458:bool, "error out"=w468:errorcluster)  [unwired: 6 in, 1 out]
                n400 = Path To String(path=w465) -> (string=w464:string)
                n401 = Search/Split String(string=w464, search string/char (-)=w463) -> (offset of match=w462:i32)  [unwired: 1 in, 2 out]
                n402 = Equal?(x=w462, y=-1) -> (x = y?=w459:bool)
                n403 = Not(x=w458) -> (.not. x?=w460:bool)
                n404 = And(x=w459, y=w460) -> (x .and. y?=w457:bool)
                n405 = case shown="False" w457 {
                  tunnel: w468 -> [w475 _]
                  tunnel: w458 -> [w474 _]
                  tunnel: w465 -> [w473 _]
                  frame False {
                    n406 = case shown="False" w474 {
                      tunnel: w475 -> [w477 _]
                      tunnel: w473 -> [w476 _]
                      frame False {
                        n407 = call "Carica specifica da file.vi"("error in (no error)"=w477, "file path"=w476) -> ()  [unwired: 4 in, 2 out]
                      }
                      frame True {
                      }
                    }
                  }
                  frame True {
                    n408 = One Button Dialog(message="IL FILE SELEZIONATO\nE' DI UN ALTRO PRODOTTO!") -> ()  [unwired: 1 in, 1 out]
                  }
                }
              }
              frame #1 {
                n409 = global read "Globali.vi" "NOME PRODOTTO"() -> (w543:string)
                n410 = global read "Globali.vi" "8. 0"() -> (w542:i16)
                n411 = global read "Globali.vi" "12. 0"() -> (w541:sgl)
                n412 = global read "Globali.vi" "16. 0"() -> (w540:i16)
                n413 = global read "Globali.vi" "20. 0"() -> (w539:u16)
                n414 = global read "Globali.vi" "22. 0"() -> (w538:sgl)
                n415 = global read "Globali.vi" "26. 0"() -> (w537:sgl)
                n416 = global read "Globali.vi" "30. 0"() -> (w536:u16)
                n417 = global read "Globali.vi" "32. 0"() -> (w535:sgl)
                n418 = global read "Globali.vi" "36. 0"() -> (w534:sgl)
                n419 = global read "Globali.vi" "40. 0"() -> (w533:u16)
                n420 = global read "Globali.vi" "42. 0"() -> (w532:u16)
                n421 = global read "Globali.vi" "44. 0"() -> (w531:i16)
                n422 = global read "Globali.vi" "48. 0"() -> (w530:u16)
                n423 = global read "Globali.vi" "50. 0"() -> (w529:i16)
                n424 = global read "Globali.vi" "54. 0"() -> (w528:u16)
                n425 = global read "Globali.vi" "56. 0"() -> (w527:i16)
                n426 = local write "12. 0"(w541) -> ()
                n427 = local write "16. 0"(w540) -> ()
                n428 = local write "20. 0"(w539) -> ()
                n429 = local write "22. 0"(w538) -> ()
                n430 = local write "26. 0"(w537) -> ()
                n431 = local write "30. 0"(w536) -> ()
                n432 = local write "32. 0"(w535) -> ()
                n433 = local write "36. 0"(w534) -> ()
                n434 = local write "40. 0"(w533) -> ()
                n435 = local write "42. 0"(w532) -> ()
                n436 = local write "44. 0"(w531) -> ()
                n437 = local write "48. 0"(w530) -> ()
                n438 = local write "50. 0"(w529) -> ()
                n439 = local write "54. 0"(w528) -> ()
                n440 = local write "56. 0"(w527) -> ()
                n441 = local write "8. 0"(w542) -> ()
                n442 = global read "Globali.vi" "60. 0"() -> (w526:u16)
                n443 = global read "Globali.vi" "62. 0"() -> (w525:i16)
                n444 = global read "Globali.vi" "66. 0"() -> (w524:u16)
                n445 = global read "Globali.vi" "68. 0"() -> (w523:i16)
                n446 = global read "Globali.vi" "72. 0"() -> (w522:sgl)
                n447 = global read "Globali.vi" "76. 0"() -> (w521:sgl)
                n448 = global read "Globali.vi" "80. 0"() -> (w520:sgl)
                n449 = global read "Globali.vi" "84. 0"() -> (w519:i16)
                n450 = global read "Globali.vi" "88. 0"() -> (w518:sgl)
                n451 = global read "Globali.vi" "92. 0"() -> (w517:sgl)
                n452 = global read "Globali.vi" "96. 0"() -> (w516:sgl)
                n453 = global read "Globali.vi" "100. 0"() -> (w515:i16)
                n454 = global read "Globali.vi" "104. 0"() -> (w514:sgl)
                n455 = global read "Globali.vi" "108. 0"() -> (w513:sgl)
                n456 = global read "Globali.vi" "112. 0"() -> (w512:sgl)
                n457 = global read "Globali.vi" "116. 0"() -> (w511:i16)
                n458 = local write "NOME PRODOTTO"(w543) -> ()
                n459 = local write "100. 0"(w515) -> ()
                n460 = local write "104. 0"(w514) -> ()
                n461 = local write "108. 0"(w513) -> ()
                n462 = local write "112. 0"(w512) -> ()
                n463 = local write "116. 0"(w511) -> ()
                n464 = local write "60. 0"(w526) -> ()
                n465 = local write "62. 0"(w525) -> ()
                n466 = local write "66. 0"(w524) -> ()
                n467 = local write "68. 0"(w523) -> ()
                n468 = local write "72. 0"(w522) -> ()
                n469 = local write "76. 0"(w521) -> ()
                n470 = local write "80. 0"(w520) -> ()
                n471 = local write "84. 0"(w519) -> ()
                n472 = local write "88. 0"(w518) -> ()
                n473 = local write "92. 0"(w517) -> ()
                n474 = local write "96. 0"(w516) -> ()
                n475 = global read "Globali.vi" "120. 0"() -> (w510:sgl)
                n476 = global read "Globali.vi" "124. 0"() -> (w509:sgl)
                n477 = global read "Globali.vi" "128. 0"() -> (w508:sgl)
                n478 = global read "Globali.vi" "132. 0"() -> (w507:u16)
                n479 = global read "Globali.vi" "134. 0"() -> (w506:sgl)
                n480 = global read "Globali.vi" "138. 0"() -> (w505:sgl)
                n481 = global read "Globali.vi" "142. 0"() -> (w504:u16)
                n482 = global read "Globali.vi" "144. 0"() -> (w503:i16)
                n483 = global read "Globali.vi" "148. 0"() -> (w502:i16)
                n484 = global read "Globali.vi" "152. 0"() -> (w501:u16)
                n485 = global read "Globali.vi" "154. 0"() -> (w500:i16)
                n486 = global read "Globali.vi" "158. 0"() -> (w499:u16)
                n487 = global read "Globali.vi" "160. 0"() -> (w498:sgl)
                n488 = global read "Globali.vi" "164. 0"() -> (w497:sgl)
                n489 = global read "Globali.vi" "168. 0"() -> (w496:sgl)
                n490 = global read "Globali.vi" "172. 0"() -> (w495:i16)
                n491 = local write "120. 0"(w510) -> ()
                n492 = local write "124. 0"(w509) -> ()
                n493 = local write "128. 0"(w508) -> ()
                n494 = local write "132. 0"(w507) -> ()
                n495 = local write "134. 0"(w506) -> ()
                n496 = local write "138. 0"(w505) -> ()
                n497 = local write "142. 0"(w504) -> ()
                n498 = local write "144. 0"(w503) -> ()
                n499 = local write "148. 0"(w502) -> ()
                n500 = local write "152. 0"(w501) -> ()
                n501 = local write "154. 0"(w500) -> ()
                n502 = local write "158. 0"(w499) -> ()
                n503 = local write "160. 0"(w498) -> ()
                n504 = local write "164. 0"(w497) -> ()
                n505 = local write "168. 0"(w496) -> ()
                n506 = local write "172. 0"(w495) -> ()
                n507 = global read "Globali.vi" "176. 0"() -> (w494:sgl)
                n508 = global read "Globali.vi" "180. 0"() -> (w493:sgl)
                n509 = global read "Globali.vi" "184. 0"() -> (w492:sgl)
                n510 = global read "Globali.vi" "188. 0"() -> (w491:u16)
                n511 = global read "Globali.vi" "190. 0"() -> (w490:sgl)
                n512 = global read "Globali.vi" "194. 0"() -> (w489:sgl)
                n513 = global read "Globali.vi" "198. 0"() -> (w488:u16)
                n514 = global read "Globali.vi" "200. 0"() -> (w487:i16)
                n515 = global read "Globali.vi" "204. 0"() -> (w486:u16)
                n516 = global read "Globali.vi" "206. 0"() -> (w485:i16)
                n517 = global read "Globali.vi" "210. 0"() -> (w484:u16)
                n518 = global read "Globali.vi" "212. 0"() -> (w483:i16)
                n519 = global read "Globali.vi" "216. 0"() -> (w482:u16)
                n520 = global read "Globali.vi" "218. 0"() -> (w481:u16)
                n521 = global read "Globali.vi" "226. 0"() -> (w479:sgl)
                n522 = global read "Globali.vi" "230. 0"() -> (w480:sgl)
                n523 = local write "176. 0"(w494) -> ()
                n524 = local write "180. 0"(w493) -> ()
                n525 = local write "184. 0"(w492) -> ()
                n526 = local write "188. 0"(w491) -> ()
                n527 = local write "190. 0"(w490) -> ()
                n528 = local write "194. 0"(w489) -> ()
                n529 = local write "198. 0"(w488) -> ()
                n530 = local write "200. 0"(w487) -> ()
                n531 = local write "204. 0"(w486) -> ()
                n532 = local write "206. 0"(w485) -> ()
                n533 = local write "210. 0"(w484) -> ()
                n534 = local write "212. 0"(w483) -> ()
                n535 = local write "216. 0"(w482) -> ()
                n536 = local write "218. 0"(w481) -> ()
                n537 = local write "226. 0"(w479) -> ()
                n538 = local write "230. 0"(w480) -> ()
              }
            }
          }
        }
        n539 = local read "8. 0"() -> (w239:i16)
        n540 = local read "80. 0"() -> (w238:sgl)
        n541 = local read "84. 0"() -> (w234:i16)
        n542 = local read "88. 0"() -> (w235:sgl)
        n543 = local read "92. 0"() -> (w226:sgl)
        n544 = local read "96. 0"() -> (w227:sgl)
        n545 = local read "100. 0"() -> (w231:i16)
        n546 = local read "104. 0"() -> (w230:sgl)
        n547 = local read "108. 0"() -> (w210:sgl)
        n548 = local read "112. 0"() -> (w211:sgl)
        n549 = local read "116. 0"() -> (w215:i16)
        n550 = local read "12. 0"() -> (w214:sgl)
        n551 = local read "120. 0"() -> (w223:sgl)
        n552 = local read "124. 0"() -> (w222:sgl)
        n553 = local read "128. 0"() -> (w218:sgl)
        n554 = local read "132. 0"() -> (w219:u16)
        n555 = Not Equal To 0?(x=w239) -> (x != 0?=w240:bool)
        n556 = Not Equal To 0?(x=w238) -> (x != 0?=w237:bool)
        n557 = Not Equal To 0?(x=w234) -> (x != 0?=w233:bool)
        n558 = Not Equal To 0?(x=w235) -> (x != 0?=w236:bool)
        n559 = Not Equal To 0?(x=w226) -> (x != 0?=w225:bool)
        n560 = Not Equal To 0?(x=w227) -> (x != 0?=w228:bool)
        n561 = Not Equal To 0?(x=w231) -> (x != 0?=w232:bool)
        n562 = Not Equal To 0?(x=w230) -> (x != 0?=w229:bool)
        n563 = Not Equal To 0?(x=w210) -> (x != 0?=w209:bool)
        n564 = Not Equal To 0?(x=w211) -> (x != 0?=w212:bool)
        n565 = Not Equal To 0?(x=w215) -> (x != 0?=w216:bool)
        n566 = Not Equal To 0?(x=w214) -> (x != 0?=w213:bool)
        n567 = Not Equal To 0?(x=w223) -> (x != 0?=w224:bool)
        n568 = Not Equal To 0?(x=w222) -> (x != 0?=w221:bool)
        n569 = Not Equal To 0?(x=w218) -> (x != 0?=w217:bool)
        n570 = Not Equal To 0?(x=w219) -> (x != 0?=w220:bool)
        n571 = property on="8. 0" class="DigNum (strict)"("Visible"=w240) -> ()  [unwired: 2 in, 2 out]
        n572 = property on="80. 0" class="DigNum (strict)"("Visible"=w237) -> ()  [unwired: 2 in, 2 out]
        n573 = property on="84. 0" class="DigNum (strict)"("Visible"=w233) -> ()  [unwired: 2 in, 2 out]
        n574 = property on="88. 0" class="DigNum (strict)"("Visible"=w236) -> ()  [unwired: 2 in, 2 out]
        n575 = property on="92. 0" class="DigNum (strict)"("Visible"=w225) -> ()  [unwired: 2 in, 2 out]
        n576 = property on="96. 0" class="DigNum (strict)"("Visible"=w228) -> ()  [unwired: 2 in, 2 out]
        n577 = property on="100. 0" class="DigNum (strict)"("Visible"=w232) -> ()  [unwired: 2 in, 2 out]
        n578 = property on="104. 0" class="DigNum (strict)"("Visible"=w229) -> ()  [unwired: 2 in, 2 out]
        n579 = property on="108. 0" class="DigNum (strict)"("Visible"=w209) -> ()  [unwired: 2 in, 2 out]
        n580 = property on="112. 0" class="DigNum (strict)"("Visible"=w212) -> ()  [unwired: 2 in, 2 out]
        n581 = property on="116. 0" class="DigNum (strict)"("Visible"=w216) -> ()  [unwired: 2 in, 2 out]
        n582 = property on="12. 0" class="DigNum (strict)"("Visible"=w213) -> ()  [unwired: 2 in, 2 out]
        n583 = property on="120. 0" class="DigNum (strict)"("Visible"=w224) -> ()  [unwired: 2 in, 2 out]
        n584 = property on="124. 0" class="DigNum (strict)"("Visible"=w221) -> ()  [unwired: 2 in, 2 out]
        n585 = property on="128. 0" class="DigNum (strict)"("Visible"=w217) -> ()  [unwired: 2 in, 2 out]
        n586 = property on="132. 0" class="DigNum (strict)"("Visible"=w220) -> ()  [unwired: 2 in, 2 out]
        n587 = local read "134. 0"() -> (w178:sgl)
        n588 = local read "138. 0"() -> (w179:sgl)
        n589 = local read "142. 0"() -> (w183:u16)
        n590 = local read "144. 0"() -> (w182:i16)
        n591 = local read "148. 0"() -> (w191:i16)
        n592 = local read "152. 0"() -> (w190:u16)
        n593 = local read "154. 0"() -> (w186:i16)
        n594 = local read "158. 0"() -> (w187:u16)
        n595 = local read "16. 0"() -> (w207:i16)
        n596 = local read "160. 0"() -> (w206:sgl)
        n597 = local read "164. 0"() -> (w202:sgl)
        n598 = local read "168. 0"() -> (w203:sgl)
        n599 = local read "172. 0"() -> (w194:i16)
        n600 = local read "176. 0"() -> (w195:sgl)
        n601 = local read "180. 0"() -> (w199:sgl)
        n602 = local read "184. 0"() -> (w198:sgl)
        n603 = Not Equal To 0?(x=w178) -> (x != 0?=w177:bool)
        n604 = Not Equal To 0?(x=w179) -> (x != 0?=w180:bool)
        n605 = Not Equal To 0?(x=w183) -> (x != 0?=w184:bool)
        n606 = Not Equal To 0?(x=w182) -> (x != 0?=w181:bool)
        n607 = Not Equal To 0?(x=w191) -> (x != 0?=w192:bool)
        n608 = Not Equal To 0?(x=w190) -> (x != 0?=w189:bool)
        n609 = Not Equal To 0?(x=w186) -> (x != 0?=w185:bool)
        n610 = Not Equal To 0?(x=w187) -> (x != 0?=w188:bool)
        n611 = Not Equal To 0?(x=w207) -> (x != 0?=w208:bool)
        n612 = Not Equal To 0?(x=w206) -> (x != 0?=w205:bool)
        n613 = Not Equal To 0?(x=w202) -> (x != 0?=w201:bool)
        n614 = Not Equal To 0?(x=w203) -> (x != 0?=w204:bool)
        n615 = Not Equal To 0?(x=w194) -> (x != 0?=w193:bool)
        n616 = Not Equal To 0?(x=w195) -> (x != 0?=w196:bool)
        n617 = Not Equal To 0?(x=w199) -> (x != 0?=w200:bool)
        n618 = Not Equal To 0?(x=w198) -> (x != 0?=w197:bool)
        n619 = property on="134. 0" class="DigNum (strict)"("Visible"=w177) -> ()  [unwired: 2 in, 2 out]
        n620 = property on="138. 0" class="DigNum (strict)"("Visible"=w180) -> ()  [unwired: 2 in, 2 out]
        n621 = property on="142. 0" class="DigNum (strict)"("Visible"=w184) -> ()  [unwired: 2 in, 2 out]
        n622 = property on="144. 0" class="DigNum (strict)"("Visible"=w181) -> ()  [unwired: 2 in, 2 out]
        n623 = property on="148. 0" class="DigNum (strict)"("Visible"=w192) -> ()  [unwired: 2 in, 2 out]
        n624 = property on="152. 0" class="DigNum (strict)"("Visible"=w189) -> ()  [unwired: 2 in, 2 out]
        n625 = property on="154. 0" class="DigNum (strict)"("Visible"=w185) -> ()  [unwired: 2 in, 2 out]
        n626 = property on="158. 0" class="DigNum (strict)"("Visible"=w188) -> ()  [unwired: 2 in, 2 out]
        n627 = property on="16. 0" class="DigNum (strict)"("Visible"=w208) -> ()  [unwired: 2 in, 2 out]
        n628 = property on="160. 0" class="DigNum (strict)"("Visible"=w205) -> ()  [unwired: 2 in, 2 out]
        n629 = property on="164. 0" class="DigNum (strict)"("Visible"=w201) -> ()  [unwired: 2 in, 2 out]
        n630 = property on="168. 0" class="DigNum (strict)"("Visible"=w204) -> ()  [unwired: 2 in, 2 out]
        n631 = property on="172. 0" class="DigNum (strict)"("Visible"=w193) -> ()  [unwired: 2 in, 2 out]
        n632 = property on="176. 0" class="DigNum (strict)"("Visible"=w196) -> ()  [unwired: 2 in, 2 out]
        n633 = property on="180. 0" class="DigNum (strict)"("Visible"=w200) -> ()  [unwired: 2 in, 2 out]
        n634 = property on="184. 0" class="DigNum (strict)"("Visible"=w197) -> ()  [unwired: 2 in, 2 out]
        n635 = local read "188. 0"() -> (w175:u16)
        n636 = local read "190. 0"() -> (w174:sgl)
        n637 = local read "194. 0"() -> (w170:sgl)
        n638 = local read "198. 0"() -> (w171:u16)
        n639 = local read "20. 0"() -> (w162:u16)
        n640 = local read "200. 0"() -> (w163:i16)
        n641 = local read "204. 0"() -> (w167:u16)
        n642 = local read "206. 0"() -> (w166:i16)
        n643 = local read "210. 0"() -> (w151:u16)
        n644 = local read "212. 0"() -> (w152:i16)
        n645 = local read "216. 0"() -> (w156:u16)
        n646 = local read "218. 0"() -> (w155:u16)
        n647 = local read "22. 0"() -> (w159:sgl)
        n648 = local read "26. 0"() -> (w158:sgl)
        n649 = local read "30. 0"() -> (w118:u16)
        n650 = local read "32. 0"() -> (w119:sgl)
        n651 = Not Equal To 0?(x=w175) -> (x != 0?=w176:bool)
        n652 = Not Equal To 0?(x=w174) -> (x != 0?=w173:bool)
        n653 = Not Equal To 0?(x=w170) -> (x != 0?=w169:bool)
        n654 = Not Equal To 0?(x=w171) -> (x != 0?=w172:bool)
        n655 = Not Equal To 0?(x=w162) -> (x != 0?=w161:bool)
        n656 = Not Equal To 0?(x=w163) -> (x != 0?=w164:bool)
        n657 = Not Equal To 0?(x=w167) -> (x != 0?=w168:bool)
        n658 = Not Equal To 0?(x=w166) -> (x != 0?=w165:bool)
        n659 = Not Equal To 0?(x=w151) -> (x != 0?=w150:bool)
        n660 = Not Equal To 0?(x=w152) -> (x != 0?=w153:bool)
        n661 = Not Equal To 0?(x=w156) -> (x != 0?=w157:bool)
        n662 = Not Equal To 0?(x=w155) -> (x != 0?=w154:bool)
        n663 = Not Equal To 0?(x=w159) -> (x != 0?=w160:bool)
        n664 = Not Equal To 0?(x=w158) -> (x != 0?=w149:bool)
        n665 = Not Equal To 0?(x=w118) -> (x != 0?=w117:bool)
        n666 = Not Equal To 0?(x=w119) -> (x != 0?=w120:bool)
        n667 = property on="188. 0" class="DigNum (strict)"("Visible"=w176) -> ()  [unwired: 2 in, 2 out]
        n668 = property on="190. 0" class="DigNum (strict)"("Visible"=w173) -> ()  [unwired: 2 in, 2 out]
        n669 = property on="194. 0" class="DigNum (strict)"("Visible"=w169) -> ()  [unwired: 2 in, 2 out]
        n670 = property on="198. 0" class="DigNum (strict)"("Visible"=w172) -> ()  [unwired: 2 in, 2 out]
        n671 = property on="20. 0" class="DigNum (strict)"("Visible"=w161) -> ()  [unwired: 2 in, 2 out]
        n672 = property on="200. 0" class="DigNum (strict)"("Visible"=w164) -> ()  [unwired: 2 in, 2 out]
        n673 = property on="204. 0" class="DigNum (strict)"("Visible"=w168) -> ()  [unwired: 2 in, 2 out]
        n674 = property on="206. 0" class="DigNum (strict)"("Visible"=w165) -> ()  [unwired: 2 in, 2 out]
        n675 = property on="210. 0" class="DigNum (strict)"("Visible"=w150) -> ()  [unwired: 2 in, 2 out]
        n676 = property on="212. 0" class="DigNum (strict)"("Visible"=w153) -> ()  [unwired: 2 in, 2 out]
        n677 = property on="216. 0" class="DigNum (strict)"("Visible"=w157) -> ()  [unwired: 2 in, 2 out]
        n678 = property on="218. 0" class="DigNum (strict)"("Visible"=w154) -> ()  [unwired: 2 in, 2 out]
        n679 = property on="22. 0" class="DigNum (strict)"("Visible"=w160) -> ()  [unwired: 2 in, 2 out]
        n680 = property on="26. 0" class="DigNum (strict)"("Visible"=w149) -> ()  [unwired: 2 in, 2 out]
        n681 = property on="30. 0" class="DigNum (strict)"("Visible"=w117) -> ()  [unwired: 2 in, 2 out]
        n682 = property on="32. 0" class="DigNum (strict)"("Visible"=w120) -> ()  [unwired: 2 in, 2 out]
        n683 = local read "36. 0"() -> (w122:sgl)
        n684 = local read "40. 0"() -> (w123:u16)
        n685 = local read "42. 0"() -> (w127:u16)
        n686 = local read "44. 0"() -> (w126:i16)
        n687 = local read "48. 0"() -> (w135:u16)
        n688 = local read "50. 0"() -> (w134:i16)
        n689 = local read "54. 0"() -> (w130:u16)
        n690 = local read "56. 0"() -> (w131:i16)
        n691 = local read "60. 0"() -> (w146:u16)
        n692 = local read "62. 0"() -> (w145:i16)
        n693 = local read "66. 0"() -> (w141:u16)
        n694 = local read "68. 0"() -> (w142:i16)
        n695 = local read "72. 0"() -> (w138:sgl)
        n696 = local read "76. 0"() -> (w139:sgl)
        n697 = local read "226. 0"() -> (w107:sgl)
        n698 = local read "230. 0"() -> (w106:sgl)
        n699 = Not Equal To 0?(x=w122) -> (x != 0?=w121:bool)
        n700 = Not Equal To 0?(x=w123) -> (x != 0?=w124:bool)
        n701 = Not Equal To 0?(x=w127) -> (x != 0?=w128:bool)
        n702 = Not Equal To 0?(x=w126) -> (x != 0?=w125:bool)
        n703 = Not Equal To 0?(x=w135) -> (x != 0?=w136:bool)
        n704 = Not Equal To 0?(x=w134) -> (x != 0?=w133:bool)
        n705 = Not Equal To 0?(x=w130) -> (x != 0?=w129:bool)
        n706 = Not Equal To 0?(x=w131) -> (x != 0?=w132:bool)
        n707 = Not Equal To 0?(x=w146) -> (x != 0?=w147:bool)
        n708 = Not Equal To 0?(x=w145) -> (x != 0?=w144:bool)
        n709 = Not Equal To 0?(x=w141) -> (x != 0?=w140:bool)
        n710 = Not Equal To 0?(x=w142) -> (x != 0?=w143:bool)
        n711 = Not Equal To 0?(x=w138) -> (x != 0?=w137:bool)
        n712 = Not Equal To 0?(x=w139) -> (x != 0?=w148:bool)
        n713 = Not Equal To 0?(x=w107) -> (x != 0?=w104:bool)
        n714 = Not Equal To 0?(x=w106) -> (x != 0?=w105:bool)
        n715 = property on="36. 0" class="DigNum (strict)"("Visible"=w121) -> ()  [unwired: 2 in, 2 out]
        n716 = property on="40. 0" class="DigNum (strict)"("Visible"=w124) -> ()  [unwired: 2 in, 2 out]
        n717 = property on="42. 0" class="DigNum (strict)"("Visible"=w128) -> ()  [unwired: 2 in, 2 out]
        n718 = property on="44. 0" class="DigNum (strict)"("Visible"=w125) -> ()  [unwired: 2 in, 2 out]
        n719 = property on="48. 0" class="DigNum (strict)"("Visible"=w136) -> ()  [unwired: 2 in, 2 out]
        n720 = property on="50. 0" class="DigNum (strict)"("Visible"=w133) -> ()  [unwired: 2 in, 2 out]
        n721 = property on="54. 0" class="DigNum (strict)"("Visible"=w129) -> ()  [unwired: 2 in, 2 out]
        n722 = property on="56. 0" class="DigNum (strict)"("Visible"=w132) -> ()  [unwired: 2 in, 2 out]
        n723 = property on="60. 0" class="DigNum (strict)"("Visible"=w147) -> ()  [unwired: 2 in, 2 out]
        n724 = property on="62. 0" class="DigNum (strict)"("Visible"=w144) -> ()  [unwired: 2 in, 2 out]
        n725 = property on="66. 0" class="DigNum (strict)"("Visible"=w140) -> ()  [unwired: 2 in, 2 out]
        n726 = property on="68. 0" class="DigNum (strict)"("Visible"=w143) -> ()  [unwired: 2 in, 2 out]
        n727 = property on="72. 0" class="DigNum (strict)"("Visible"=w137) -> ()  [unwired: 2 in, 2 out]
        n728 = property on="76. 0" class="DigNum (strict)"("Visible"=w148) -> ()  [unwired: 2 in, 2 out]
        n729 = property on="226. 0" class="DigNum (strict)"("Visible"=w104) -> ()  [unwired: 2 in, 2 out]
        n730 = property on="230. 0" class="DigNum (strict)"("Visible"=w105) -> ()  [unwired: 2 in, 2 out]
      }
    }
  }
  n731 = call "Carica immagine.vi"("Immagine JPG"="Logo cliente.jpg") -> ("altezza"=w20:i16, "larghezza"=w21:i16, "Picture"=→"Picture":picture)  [unwired: 2 in]
  n732 = call "Leggi file testi.vi"("Numero riga"=0) -> ("Testo"=→"Linea":string)  [unwired: 3 in, 1 out]
  n733 = Bundle("larghezza"=w21, "altezza"=w20) -> (w19:cluster{"larghezza":i16, "altezza":i16})  [unwired: 1 in]
  n734 = property on="Linea" class="Str"("Disabled"=u8 1) -> ()  [unwired: 2 in, 2 out]
  n735 = property on="Picture" class="Pict"("Draw Area Size"=w19) -> ()  [unwired: 2 in, 2 out]
  n736 = global read "Globali.vi" "Versione SW"() -> (→"Versione SW":dbl)
  n737 = global read "Globali.vi" "Prodotto"() -> (w3:string)
  n738 = Match Pattern(string=w3, regular expression=" -") -> (before substring=→"Prodotto":string)  [unwired: 1 in, 3 out]
  n739 = global read "Globali.vi" "Indicazioni"() -> (→"Indicazioni":string)
  "Tipo pagina" <- "PAGINA PARAMETRI" ("Tipo pagina")
